vi "Untitled 1.vi"() -> ()   [LabVIEW 2020]
panel:
  out "Fuera de rango":bool
  in  "Stop":bool
  out "No. Muestras":i32
  in  "Limite de muestreo":i32
  in  "Limite superior":dbl
  in  "Tiempo de muestreo":dbl
  out "Fecha":string
  out "Temperatura":cluster{dbl, "Numeric":dbl}(graph)
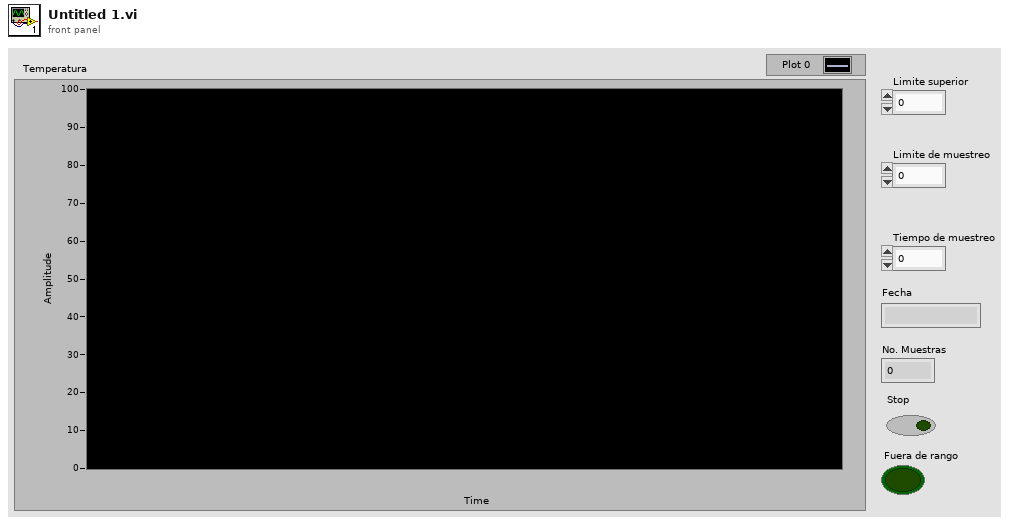
[diagram p1: front panel]
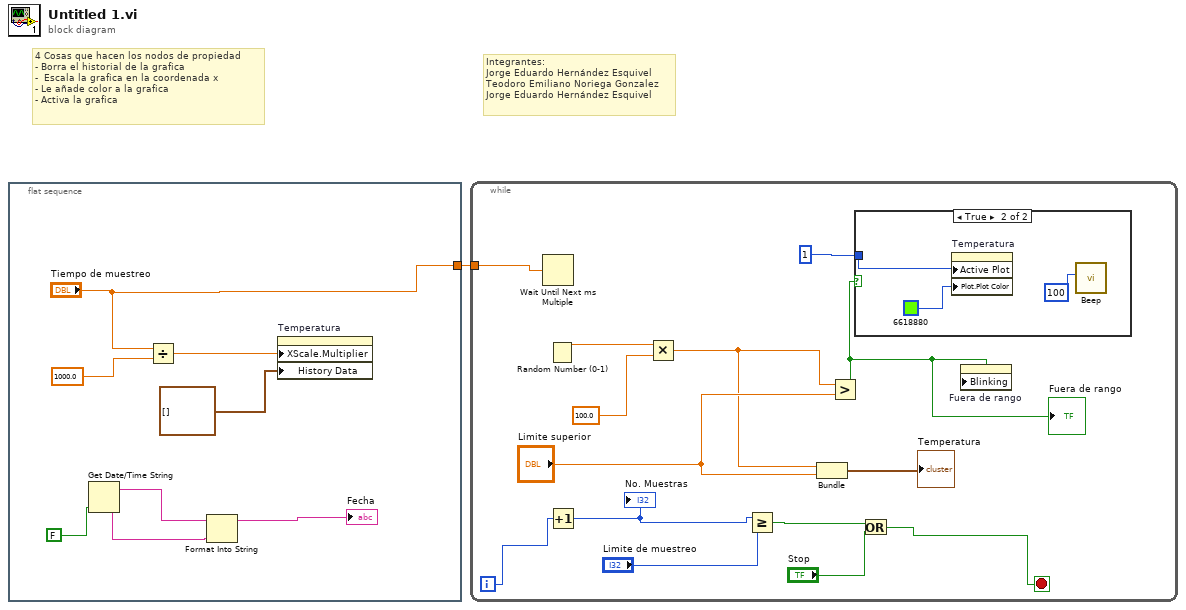
[diagram p0: block diagram]
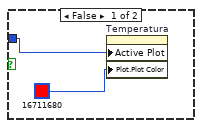
[diagram p2: hidden frame]
diagram:
  # "Integrantes:\nJorge Eduardo Hernández Esquivel\nTeodoro Emiliano Noriega Gonzalez\nJorge Eduardo Hernández Esquivel"
  # "4 Cosas que hacen los nodos de propiedad \n- Borra el historial de la grafica \n-  Escala la grafica en la coordenada x\n- Le añade color a la grafica \n- Activa la grafica"
  n1 = flat-sequence {
    tunnel: ["Tiempo de muestreo"] -> w1
    frame #0 {
      n2 = Get Date/Time String(want seconds? (F)=FALSE) -> (date string=w6:string, time string=w7:string)  [unwired: 2 in]
      n3 = Divide(x="Tiempo de muestreo", y=1000.0) -> (x/y=w4:dbl)
      n4 = Format Into String "Format Into String"(initial string=w6, w7) -> (resulting string=→"Fecha":string)  [unwired: 2 in, 1 out]
      n5 = property on="Temperatura" class="WFChart (strict)"("XScale.Multiplier"=w4, "History Data"=cluster{dbl, "Numeric":dbl}[] []) -> ()  [unwired: 2 in, 2 out]
    }
  }
  n6 = while {
    tunnel: w1 -> [w14]
    i -> [w19]
    stop <- w15 stop-if-true
    n7 = Wait Until Next ms Multiple(millisecond multiple=w14) -> ()  [unwired: 1 out]
    n8 = Random Number (0-1)() -> (number: 0 to 1=w22:dbl)
    n9 = Increment(x=w19) -> (x+1=w17:i32)
    "No. Muestras" <- w17
    n10 = Multiply(x=w22, y=100.0) -> (x*y=w20:dbl)
    n11 = Greater Or Equal?(x=w17, y="Limite de muestreo") -> (x >= y?=w16:bool)
    n12 = Bundle(w20, "Limite superior"="Limite superior") -> (→"Temperatura":cluster{dbl, "Limite superior ":dbl})  [unwired: 1 in]
    n13 = Greater?(x=w20, y="Limite superior") -> (0:w11:bool)
    "Fuera de rango" <- w11
    n14 = case shown="True" w11 {
      tunnel: 1 -> [w25 w26]
      frame False {
        n15 = property on="Temperatura" class="WFChart (strict)"("Active Plot"=w25, "Plot.Plot Color"=u32 16711680) -> ()  [unwired: 2 in, 2 out]
      }
      frame True {
        n16 = property on="Temperatura" class="WFChart (strict)"("Active Plot"=w26, "Plot.Plot Color"=u32 6618880) -> ()  [unwired: 2 in, 2 out]
        n17 = call <vilib>:"Beep.vi"("duration (msec)"=u32 100) -> ()  [unwired: 11 in]
      }
    }
    n18 = Or(x=w16, y="Stop") -> (x .or. y?=w15:bool)
    n19 = property on="Fuera de rango" class="Bool (strict)"("Blinking"=w11) -> ()  [unwired: 2 in, 2 out]
  }
